vi "Test Data Package.vi"() -> ()   [LabVIEW 2014]
uses:
  <vilib>/Analysis/Matrix/Datatypes/RealMatrix.ctl
  <vilib>/Analysis/Matrix/NI_Matrix.lvlib
  reusable/CRDS/Cell/hkParam Ctl.ctl
  reusable/CRDS/Data/Cell/CRDS Cell Data.lvclass
  reusable/CRDS/Cell/extParam Ctl.ctl
  reusable/CRDS/Data/Main/CRDS Data.lvclass
  reusable/PAS/Data/Main/PAS Data.lvclass
  reusable/PAS/Data/Cell/PAS Cell Data.lvclass
  PAS/Data/Cell/ePAS Cell Data.lvclass
panel:
  in  "data":u8
  out "length":i32
  out "String":string
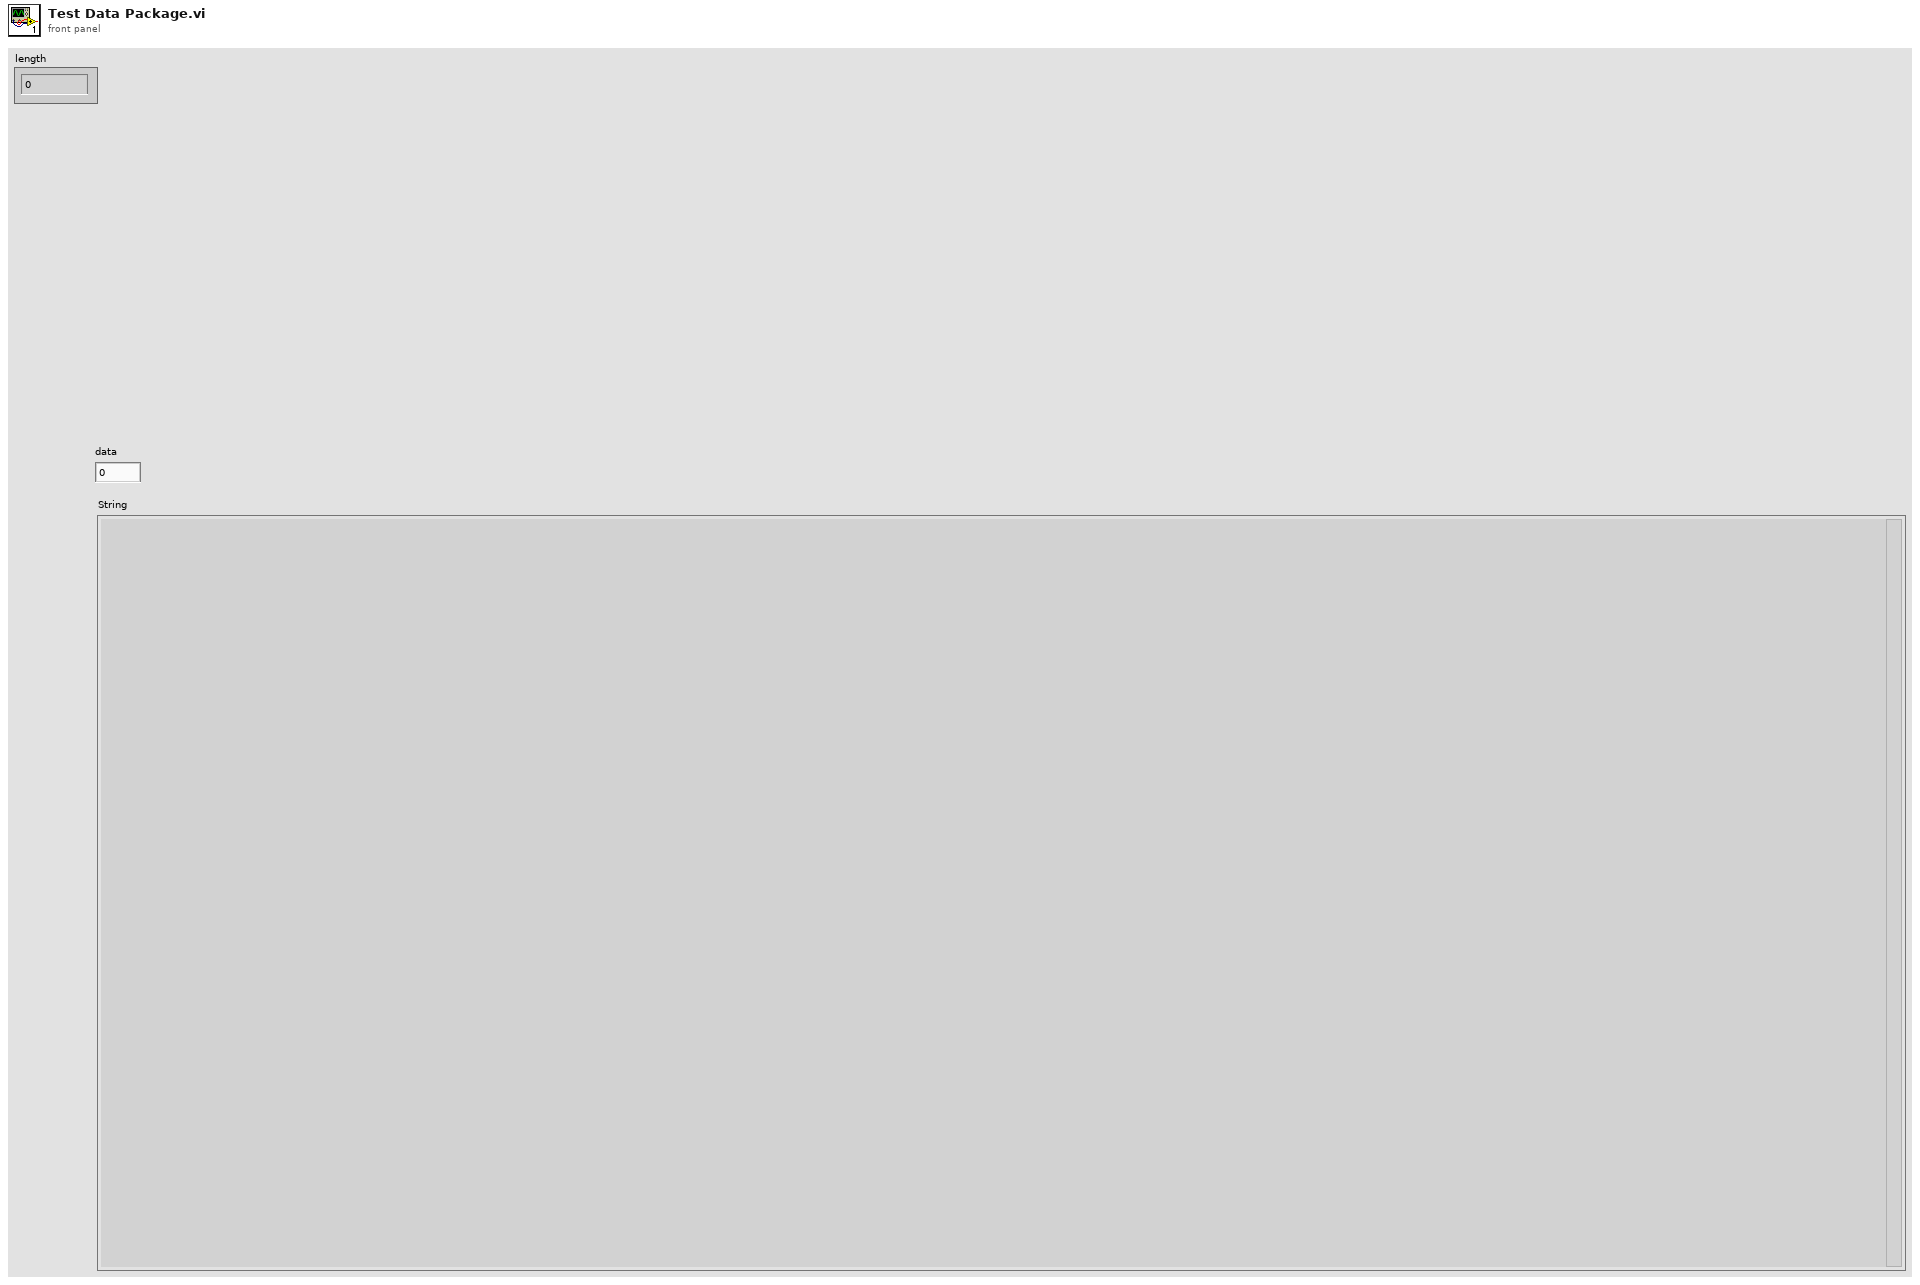
[diagram p1: front panel]
types:
  T1 = typedef "CRDS Lib.lvlib/CRDS Cell Data.lvclass/extParam Ctl.ctl" = cluster{"Tau":sgl, "Tau0cor":sgl, "ext":sgl, "extCorr":sgl, "stdevTau":sgl, "eTau":sgl, "taucorr":sgl, "Tau0":sgl, "max":sgl}
  T2 = typedef "CRDS Lib.lvlib/CRDS Cell Data.lvclass/hkParam Ctl.ctl" = cluster{"rhDilFac":sgl, "Q":sgl, "Tmean":sgl, "extDilFac":sgl, "rhCell":sgl, "P":sgl, "T":sgl}
  T3 = cluster{"AllanVar":cluster{"iTime":sgl[], "stdDev":sgl[]}, "extParam":T1, "hkData":T2, "Ringdowns":i16[][]}
  T4 = cluster{"AllanVar":cluster{"iTime":sgl[], "stdDev":sgl[]}, "extParam":T1, "hkData":T2}
  T5 = cluster{"Time":dbl, "CellData":cluster{"AllanVar":cluster{"iTime":sgl[], "stdDev":sgl[]}, "extParam":T1, "hkData":T2, "Ringdowns":i16[][]}[]}
  T6 = cluster{"Time":dbl, "CellData":cluster{"AllanVar":cluster{"iTime":sgl[], "stdDev":sgl[]}, "extParam":T1, "hkData":T2}[]}
  T7 = typedef "NI_Matrix.lvlib/RealMatrix.ctl" = dbl[][]
  T8 = cluster{"derived":cluster{"f0":sgl, "IA":sgl, "Q":sgl, "max":dbl[], "noiseLim":dbl, "ext":dbl}, "fitData":cluster{"parameters":dbl[], "covariance":T7}, "IABack":dbl}
  T9 = cluster{"Time":dbl, "Drive":bool, "CellData":cluster{"derived":cluster{"f0":sgl, "IA":sgl, "Q":sgl, "max":dbl[], "noiseLim":dbl, "ext":dbl}, "fitData":cluster{"parameters":dbl[], "covariance":T7}, "IABack":dbl}[], "FittedData":cluster{"Y":sgl[], "dt":dbl}[], "MicFreq":cluster{"Y":sgl[], "dt":dbl}[], "MicTime":cluster{"Y":i16[], "dt":dbl}[], "Photodiode":cluster{"Y":i16[], "dt":dbl}[]}
  T10 = cluster{"Time":dbl, "Drive":bool, "CellData":cluster{"derived":cluster{"f0":sgl, "IA":sgl, "Q":sgl, "max":dbl[], "noiseLim":dbl, "ext":dbl}, "fitData":cluster{"parameters":dbl[], "covariance":T7}, "IABack":dbl}[]}
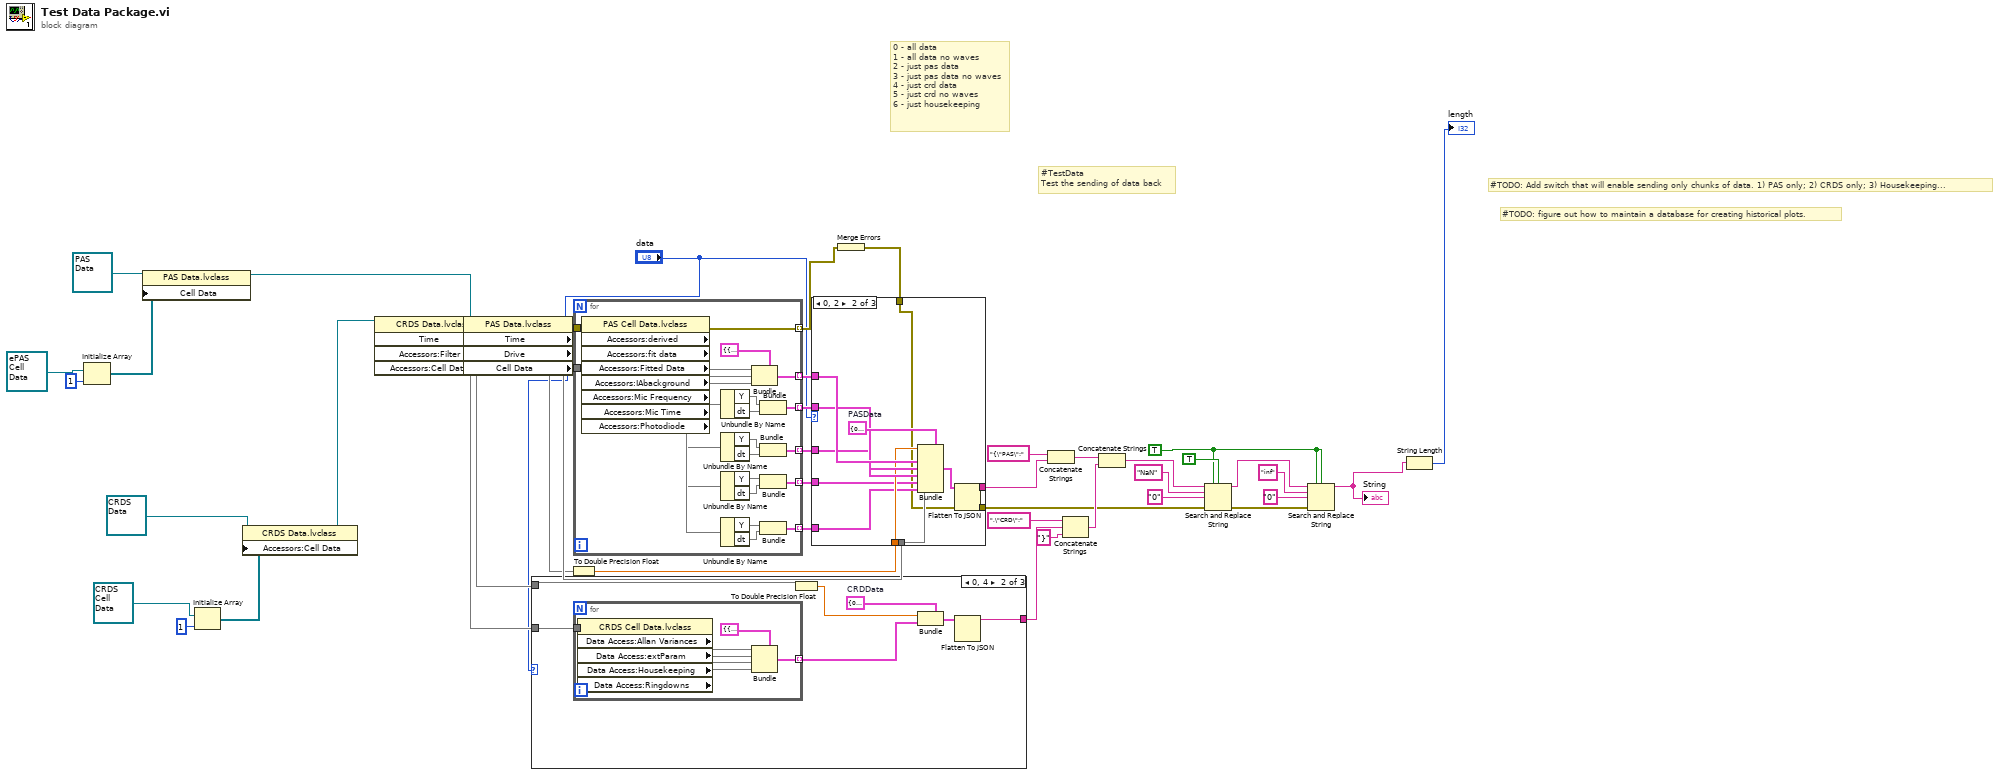
[diagram p0: block diagram]
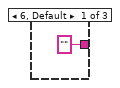
[diagram p2: hidden frame]
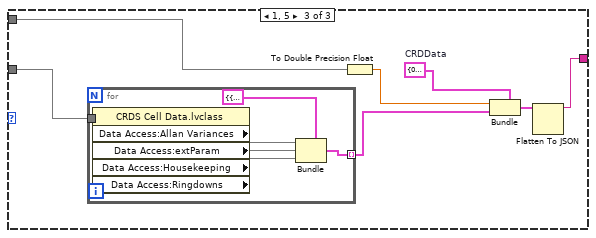
[diagram p3: hidden frame]
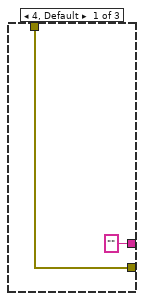
[diagram p4: hidden frame]
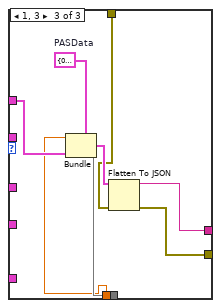
[diagram p5: hidden frame]
diagram:
  w20 = TRUE ("replace all? (F)")
  # "#TestData\nTest the sending of data back"
  # "0 - all data\n1 - all data no waves\n2 - just pas data\n3 - just pas data no waves\n4 - just crd data\n5 - just crd no waves\n6 - just housekeeping"
  # "#TODO: figure out how to maintain a database for creating historical plots."
  # "#TODO: Add switch that will enable sending only chunks of data. 1) PAS only; 2) CRDS only; 3) Housekeeping..."
  n1 = Initialize Array(refnum<class "ePAS Cell Data.lvclass"> refnum ("ePAS Cell"), 1 ("dimension size")) -> (w7:refnum<class "ePAS Cell Data.lvclass">[])
  n2 = property class="PAS Data.lvclass"(reference=refnum<class "PAS Data.lvclass"> refnum ("PAS Data"), "Cell Data"=w7) -> (reference out=w6:refnum<class "PAS Data.lvclass">)  [unwired: 1 in, 1 out]
  n3 = Initialize Array(refnum<class "CRDS Cell Data.lvclass"> refnum ("CRDS Cell"), 1 ("dimension size")) -> (w2:refnum<class "CRDS Cell Data.lvclass">[])
  n4 = property class="CRDS Data.lvclass"(reference=refnum<class "CRDS Data.lvclass"> refnum ("CRDS"), "Accessors:Cell Data"=w2) -> (reference out=w1:refnum<class "CRDS Data.lvclass">)  [unwired: 1 in, 1 out]
  n5 = property class="CRDS Data.lvclass" props=["Time", "Accessors:Filter", "Accessors:Cell Data"](reference=w1) -> (error out=w17:errorcluster, "Time"=w40, "Accessors:Cell Data"=w41)  [unwired: 1 in, 2 out]
  n6 = property class="PAS Data.lvclass"(reference=w6, error in=w17) -> (error out=w16:errorcluster, "Time"=w36, "Drive"=w43, "Cell Data"=w42)  [unwired: 1 out]
  n7 = case shown="0, 4" "data" {
    tunnel: w41 -> [_ w53 w64]
    tunnel: w40 -> [_ w49 w65]
    tunnel: ["" ("JSON string") w47 w61] -> w29
    frame 6, Default {
    }
    frame 0, 4 {
      w52 = T5 {"Time"=0.0, "CellData"=[]}  # CRDData
      n8 = for {
        tunnel: w53 -> [w60]
        tunnel: [w54] -> w51 mode=indexing
        n9 = property class="CRDS Cell Data.lvclass"(reference=w60) -> ("Data Access:Allan Variances"=w59, "Data Access:extParam"=w58, "Data Access:Housekeeping"=w57, "Data Access:Ringdowns"=w56)  [unwired: 1 in, 2 out]
        n10 = Bundle(cluster=T3 {"AllanVar"={"iTime"=[], "stdDev"=[]}, "extParam"={"Tau"=0.0, "Tau0cor"=0.0, "ext"=0.0, "extCorr"=0.0, "stdevTau"=0.0, "eTau"=0.0, "taucorr"=0.0, "Tau0"=0.0, "max"=0.0}, "hkData"={"rhDilFac"=0.0, "Q"=0.0, "Tmean"=0.0, "extDilFac"=0.0, "rhCell"=0.0, "P"=0.0, "T"=0.0}, "Ringdowns"=[]}, "AllanVar"=w59, "extParam"=w58, "hkData"=w57, "Ringdowns"=w56) -> (w54:T3)
      }
      n11 = To Double Precision Float(number=w49) -> (double precision float=w48:dbl)
      n12 = Bundle(cluster=w52, "Time"=w48, "CellData"=w51) -> (w50:T5)
      n13 = Flatten To JSON(anything=w50) -> (JSON string=w47:string)  [unwired: 2 in, 1 out]
    }
    frame 1, 5 {
      w63 = T6 {"Time"=0.0, "CellData"=[]}  # CRDData
      n14 = for {
        tunnel: w64 -> [w73]
        tunnel: [w69] -> w62 mode=indexing
        n15 = property class="CRDS Cell Data.lvclass" props=["Data Access:Allan Variances", "Data Access:extParam", "Data Access:Housekeeping", "Data Access:Ringdowns"](reference=w73) -> ("Data Access:Allan Variances"=w72, "Data Access:extParam"=w71, "Data Access:Housekeeping"=w70)  [unwired: 1 in, 3 out]
        n16 = Bundle(cluster=T4 {"AllanVar"={"iTime"=[], "stdDev"=[]}, "extParam"={"Tau"=0.0, "Tau0cor"=0.0, "ext"=0.0, "extCorr"=0.0, "stdevTau"=0.0, "eTau"=0.0, "taucorr"=0.0, "Tau0"=0.0, "max"=0.0}, "hkData"={"rhDilFac"=0.0, "Q"=0.0, "Tmean"=0.0, "extDilFac"=0.0, "rhCell"=0.0, "P"=0.0, "T"=0.0}}, "AllanVar"=w72, "extParam"=w71, "hkData"=w70) -> (w69:T4)
      }
      n17 = To Double Precision Float(number=w65) -> (double precision float=w66:dbl)
      n18 = Bundle(cluster=w63, "Time"=w66, "CellData"=w62) -> (w67:T6)
      n19 = Flatten To JSON(anything=w67) -> (JSON string=w61:string)  [unwired: 2 in, 1 out]
    }
  }
  n20 = To Double Precision Float(number=w36) -> (double precision float=w35:dbl)
  n21 = for {
    tunnel: w42 -> [w97]
    tunnel: [w94] -> w39 mode=indexing
    tunnel: [w79] -> w38 mode=indexing
    tunnel: [w78] -> w37 mode=indexing
    tunnel: [w77] -> w34 mode=indexing
    tunnel: [w76] -> w33 mode=indexing
    tunnel: w16 -> [w75]
    tunnel: [w74] -> w13 mode=indexing
    n22 = property class="PAS Cell Data.lvclass"(reference=w97, error in=w75) -> (error out=w74:errorcluster, "Accessors:derived"=w96, "Accessors:fit data"=w95, "Accessors:Fitted Data"=w83, "Accessors:IAbackground"=w80, "Accessors:Mic Frequency"=w86, "Accessors:Mic Time"=w89, "Accessors:Photodiode"=w92)  [unwired: 1 out]
    n23 = Unbundle By Name(w83) -> ("Y"=w82, "dt"=w81)
    n24 = Unbundle By Name(w86) -> ("Y"=w85, "dt"=w84)
    n25 = Unbundle By Name(w89) -> ("Y"=w88, "dt"=w87)
    n26 = Unbundle By Name(w92) -> ("Y"=w91, "dt"=w90)
    n27 = Bundle(cluster=T8 {"derived"={"f0"=0.0, "IA"=0.0, "Q"=0.0, "max"=[], "noiseLim"=0.0, "ext"=0.0}, "fitData"={"parameters"=[], "covariance"=[]}, "IABack"=0.0}, "derived"=w96, "fitData"=w95, "IABack"=w80) -> (w94:T8)
    n28 = Bundle("Y"=w82, "dt"=w81) -> (w79:cluster{"Y":void, "dt":void})  [unwired: 1 in]
    n29 = Bundle("Y"=w85, "dt"=w84) -> (w78:cluster{"Y":void, "dt":void})  [unwired: 1 in]
    n30 = Bundle("Y"=w88, "dt"=w87) -> (w77:cluster{"Y":void, "dt":void})  [unwired: 1 in]
    n31 = Bundle("Y"=w91, "dt"=w90) -> (w76:cluster{"Y":void, "dt":void})  [unwired: 1 in]
  }
  n32 = Merge Errors(w13) -> (w12:errorcluster)
  n33 = case shown="0, 2" "data" {
    tunnel: w43 -> [_ w111 w116]
    tunnel: w39 -> [_ w109 w117]
    tunnel: w38 -> [_ w108 _]
    tunnel: w37 -> [_ w107 _]
    tunnel: w35 -> [_ w105 w115]
    tunnel: w34 -> [_ w104 _]
    tunnel: w33 -> [_ w103 _]
    tunnel: ["" ("JSON string") w102 w114] -> w32
    tunnel: [w98 w101 w113] -> w15
    tunnel: w12 -> [w98 w100 w112]
    frame 4, Default {
    }
    frame 0, 2 {
      w110 = T9 {"Time"=0.0, "Drive"=FALSE, "CellData"=[], "FittedData"=[], "MicFreq"=[], "MicTime"=[], "Photodiode"=[]}  # PASData
      n34 = Bundle(cluster=w110, "Time"=w105, "Drive"=w111, "CellData"=w109, "FittedData"=w108, "MicFreq"=w107, "MicTime"=w104, "Photodiode"=w103) -> (w106:T9)
      n35 = Flatten To JSON(anything=w106, error in (no error)=w100) -> (JSON string=w102:string, 11:w101:errorcluster)  [unwired: 1 in]
    }
    frame 1, 3 {
      w118 = T10 {"Time"=0.0, "Drive"=FALSE, "CellData"=[]}  # PASData
      n36 = Bundle(cluster=w118, "Time"=w115, "Drive"=w116, "CellData"=w117) -> (w119:T10)
      n37 = Flatten To JSON(anything=w119, error in (no error)=w112) -> (JSON string=w114:string, 11:w113:errorcluster)  [unwired: 1 in]
    }
  }
  n38 = Concatenate Strings("{\"PAS\":" ("string"), w32) -> (w30:string)
  n39 = Concatenate Strings(",\"CRD\":" ("string"), w29, "}" ("string")) -> (w26:string)
  n40 = Concatenate Strings(w30, w26) -> (w25:string)
  n41 = Search and Replace String(replace all?=w20, case sensitive?=TRUE ("ignore case? (F)"), input string=w25, search string="NaN", replace string="0" ("replace string (\"\")"), error in=w15) -> (result string=w21:string, error out=w14:errorcluster)  [unwired: 2 in, 2 out]
  n42 = Search and Replace String(replace all?=w20, case sensitive?=w20, input string=w21, search string="inf", replace string="0" ("replace string (\"\")"), error in=w14) -> (result string=w44:string)  [unwired: 2 in, 3 out]
  "String" <- w44
  n43 = String Length(string=w44) -> (length=→"length":i32)
